vi "23.vi"(6 "LRU Cache Size":i32, 7 "Part 1":bool, 8 "error in (no error)":errorcluster, 9 "Sample?":bool, 10 "Sample":string="#############\n#...........#\n###A#B#D#C###\n  #A#B#C#D#\n  #########", 11 "input":path=path "C:/Users/craig.walker/Documents/GitHub/lv2019-Advent-of-Code-2021/23/input.txt") -> (0 "error out":errorcluster, 2 "Best Cost":u64)   [LabVIEW 2019, in "23.lvlib"]
uses:
  23.lvlib
  lv2019-LRU-Cache/LRU Node/LRU Node.lvclass/LRU Node.ctl
  lv2019-LRU-Cache/LRU Cache/LRU Cache.lvclass/LRU Cache.ctl
  State/Write Best Cost.vi
  State/Write Rooms.vi
  State/Write Hallway.vi
  lv2019-LRU-Cache/LRU Cache/Shutdown.vi
  lv2019-LRU-Cache/LRU Node/Read Value.vi
  lv2019-LRU-Cache/LRU Node/Write Value.vi
  lv2019-LRU-Cache/LRU Node/Read Key.vi
  lv2019-LRU-Cache/LRU Node/Write Key.vi
  State/State.lvclass
  C:/Users/craig.walker/Documents/GitHub/lv2019-LRU-Cache/LRU Node/LRU Node.lvclass
  lv2019-LRU-Cache/LRU DLL/LRU DLL.lvclass
  C:/Users/craig.walker/Documents/GitHub/lv2019-Doubly-Linked-List/Doubly Linked List/Doubly Linked List.lvclass
  <userlib>/_OpenG.lib/string/string.llb/String to Character Array__ogtk.vi
  lv2019-LRU-Cache/LRU Cache/Initialise.vi
  State/Find Best Cost Core.vi
  lv2019-Doubly-Linked-List/Doubly Linked List/Shutdown.vi
  State Key/State Key.lvclass
  State Value/State Value.lvclass
  lv2019-LRU-Cache/LRU Cache/LRU Cache.lvclass
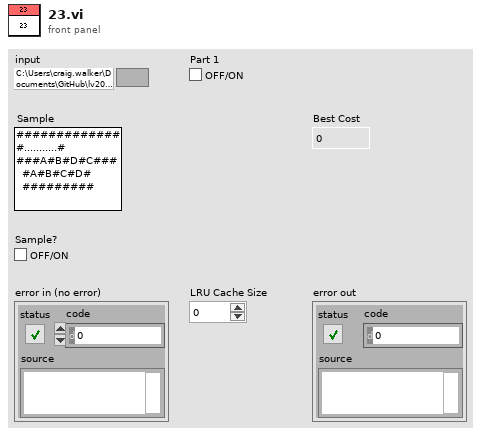
[diagram p1: front panel]
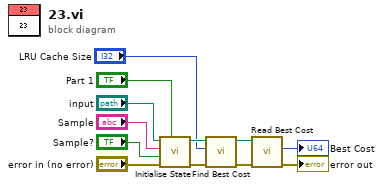
[diagram p0: block diagram]
diagram:
  n1 = call "Initialise State.vi"("Part 1?"="Part 1", "error in (no error)"="error in (no error)", "Sample?"="Sample?", "Sample"="Sample", "Input (use dialog)"="input") -> ("error out"=w9:errorcluster, "State out"=w12:refnum<class "State.lvclass">)  [unwired: 5 in]
  n2 = call "Find Best Cost.vi"("error in (no error)"=w9, "LRU Cache Size"="LRU Cache Size", "State in"=w12) -> ("error out"=w8:errorcluster, "State out"=w11:refnum<class "State.lvclass">)  [unwired: 7 in]
  n3 = call "Read Best Cost.vi"("error in (no error)"=w8, "State in"=w11) -> ("error out"=→"error out":errorcluster, "Best Cost"=→"Best Cost":u64)  [unwired: 7 in, 1 out]
